vi "PicoLog_main.vi"() -> ()   [LabVIEW 2014]
uses:
  picohrdl.dll
panel:
  in  "Save?":bool=TRUE caption="Save"
  out "noOfOpen\nChannels":i16=1
  out "Ch nr. 14":string[](array[string])
  out "Ch nr. 13":string[](array[string])
  out "Ch nr. 12":string[](array[string])
  out "Ch nr. 11":string[](array[string])
  out "Ch nr. 10":string[](array[string])
  out "Ch nr. 9":string[](array[string])
  out "Ch nr. 8":string[](array[string])
  out "Ch nr. 7":string[](array[string])
  out "Ch nr. 6":string[](array[string])
  out "Ch nr. 5":string[](array[string])
  out "Ch nr. 4":string[](array[string])
  out "Ch nr. 3":string[](array[string])
  out "Ch nr. 2.35":string[](array[string])
  out "Ch nr. 2":string[](array[string])
  out "Ch nr. 1":string[](array[string])
  out "Ch nr. 0":string[](array[string])=["1", "8"]
  out "P1 17":dbl[](graph)
  out "P1 16":dbl[](graph)
  out "P1 15":dbl[](graph)
  out "P1 14":dbl[](graph)
  out "P1 13":dbl[](graph)
  out "P1 12":dbl[](graph)
  out "P1 11":dbl[](graph)
  out "P1 10":dbl[](graph)
  out "P1 9":dbl[](graph)
  out "P1 8":dbl[](graph)
  out "P1 7":dbl[](graph)
  out "P1 6":dbl[](graph)
  out "P1 5":dbl[](graph)
  out "P1 4":dbl[](graph)
  out "P1 3":dbl[](graph)
  out "P1 2":dbl[](graph)
  in  "Voltage range":i32[](array[numeric])=[0, 0, 0, 0, 0, 0, 0, 0, 0, 0, 0, 0, 0, 0, 0, 0] min=0 max=6 step=1
  in  "Single ended\n(1- single)\n(0 - difer)":i32[](array[numeric])=[1, 1, 1, 1, 1, 1, 1, 1, 1, 1, 1, 1, 1, 1, 1, 1] min=0 max=1 step=1
  in  "Ch nr":bool[](array[boolean])=[FALSE, FALSE, FALSE, FALSE, FALSE, FALSE, FALSE, FALSE, FALSE, FALSE, FALSE, FALSE, FALSE, FALSE, FALSE, FALSE]
  in  "conversionTime":i16(ring)=3 items=["60 ms", "100 ms", "180 ms", "340 ms", "660 ms"]
  in  "Mains Frequency":i16(ring) items=["50 Hz", "60 Hz"]
  in  "sampleInterval_ms":i32=1000
  in  "stop":bool
  # "1       2       3      4       5        6       7       8       9      10     11      12     13    14       15     16"
  # "0 -+2500mV\n1 -+1250mV\n2 -+625mV\n3 -+313mV\n4 -+156mV\n5 -+78mv\n6 -+39mV"
  # "Channel"
  # "Channel"
  # "Channel"
  # "Channel"
  # "Channel"
  # "Channel"
  # "Channel"
  # "Channel"
  # "Channel"
  # "Channel"
  # "Channel"
  # "Channel"
  # "Channel"
  # "Channel"
  # "Channel"
  # "Channel"
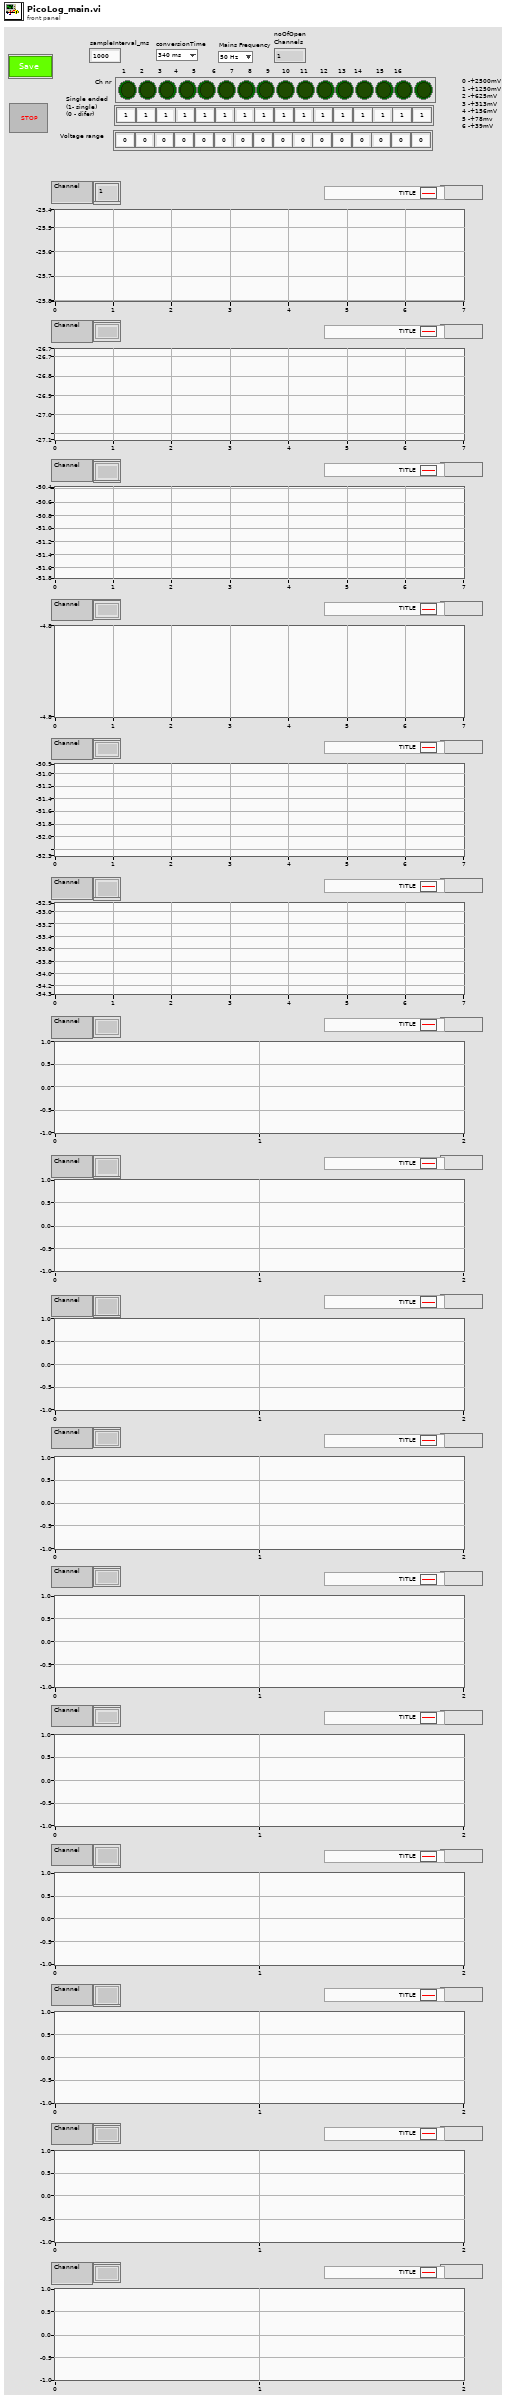
[diagram p1: front panel]
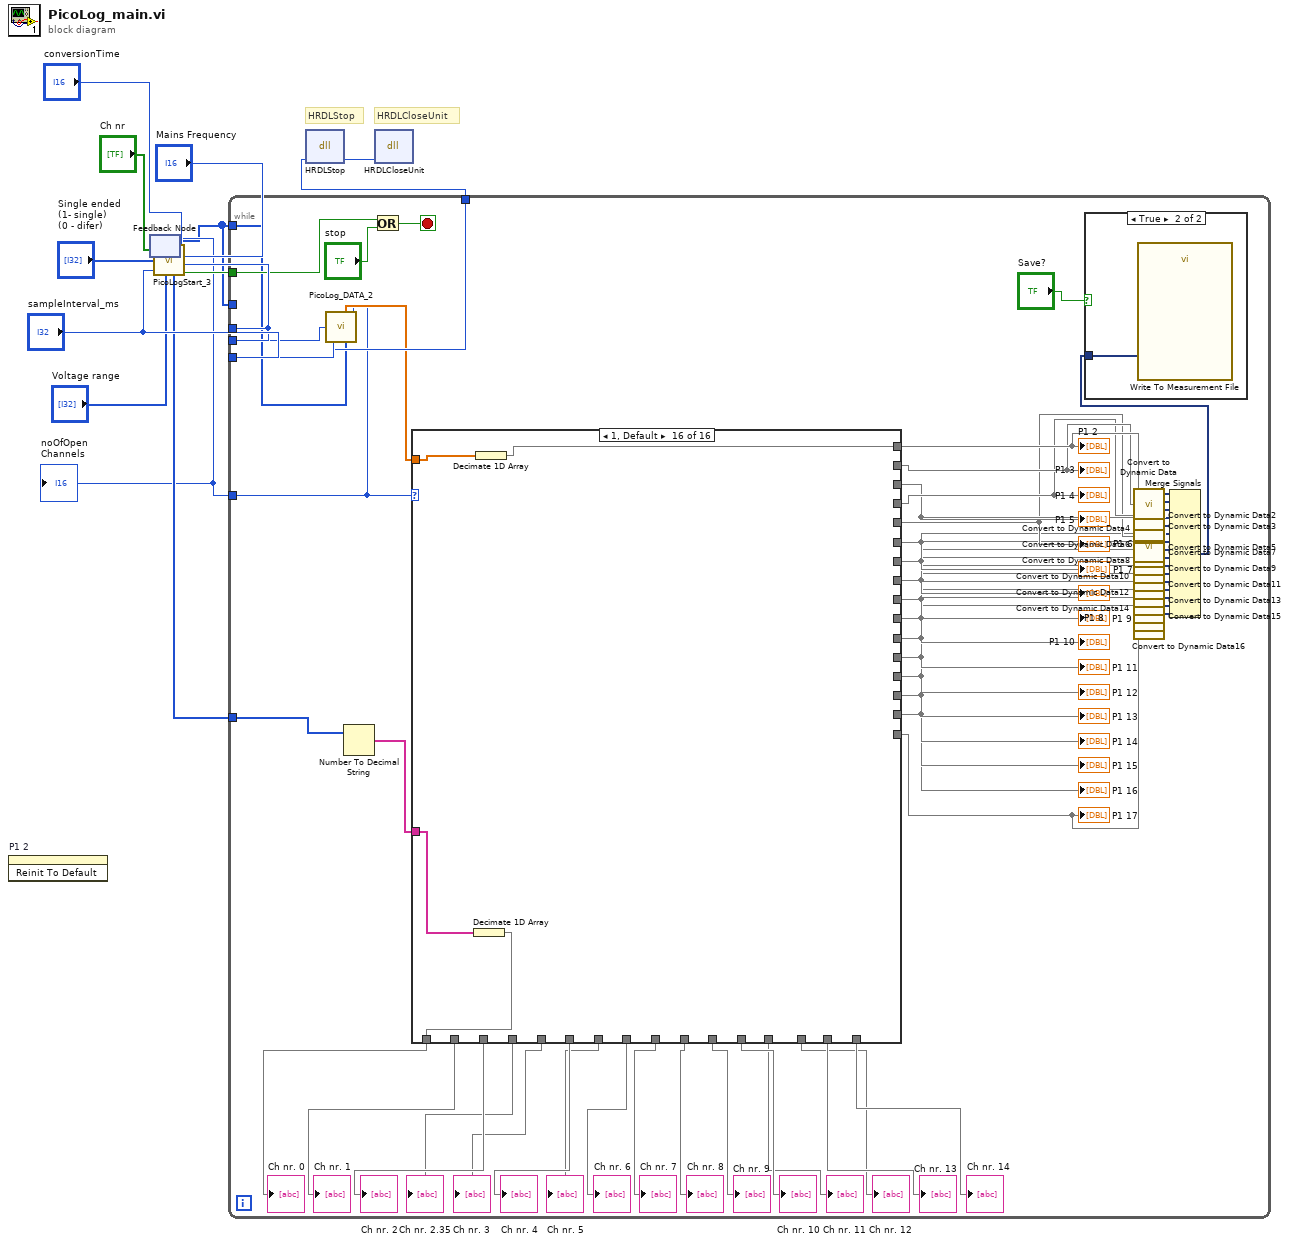
[diagram p0: block diagram]
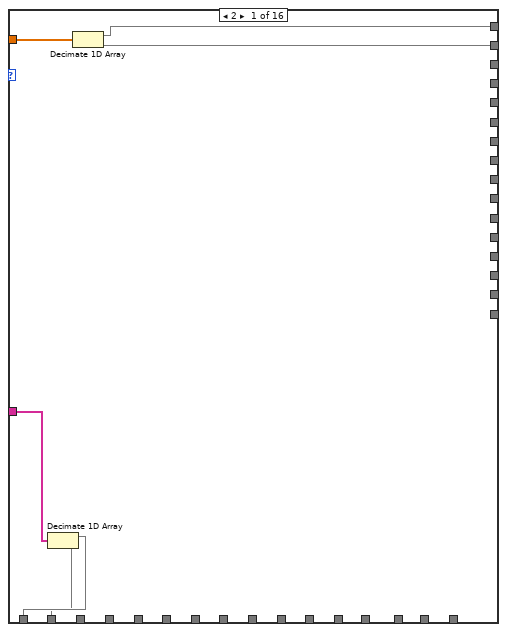
[diagram p3: hidden frame]
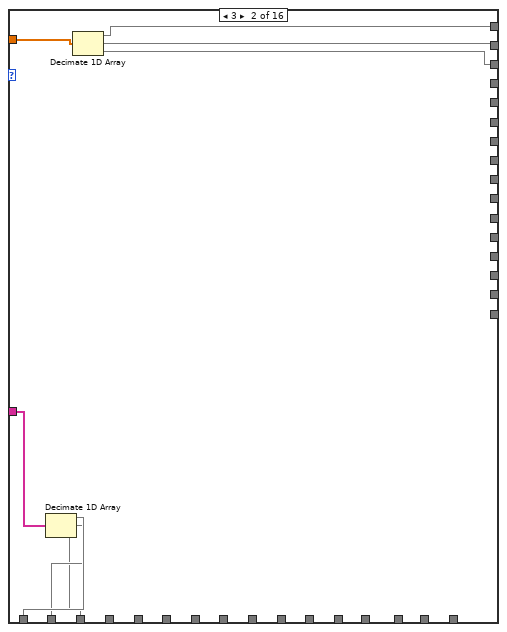
[diagram p4: hidden frame]
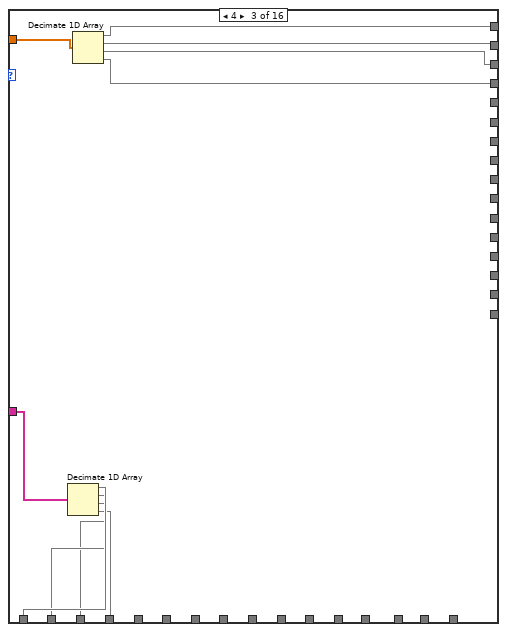
[diagram p5: hidden frame]
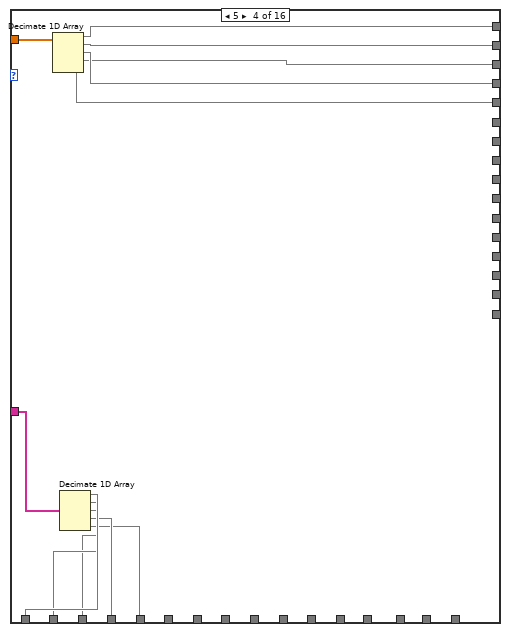
[diagram p6: hidden frame]
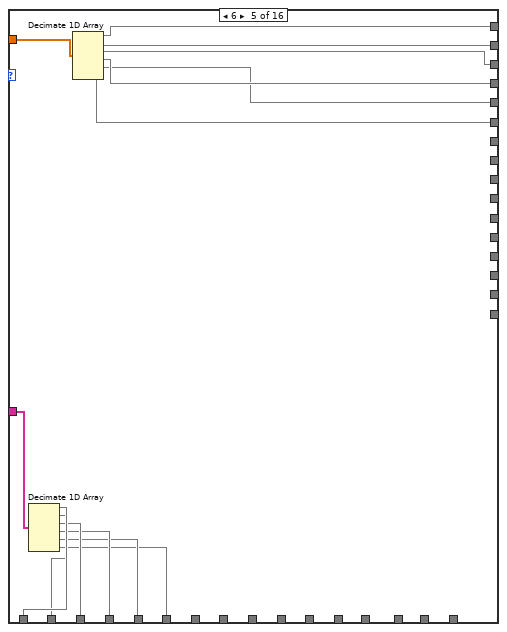
[diagram p7: hidden frame]
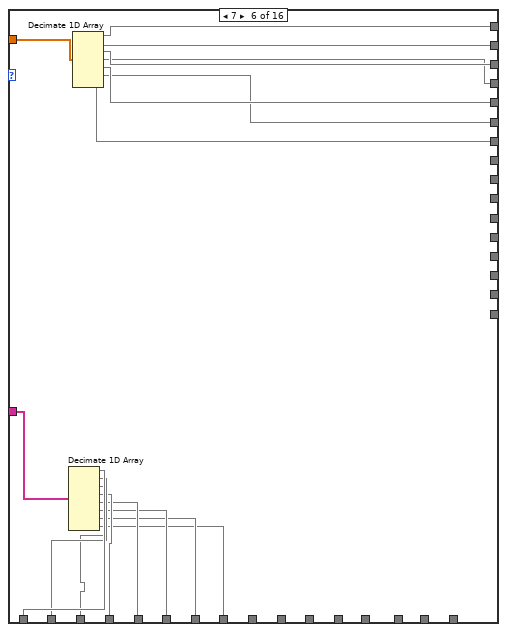
[diagram p8: hidden frame]
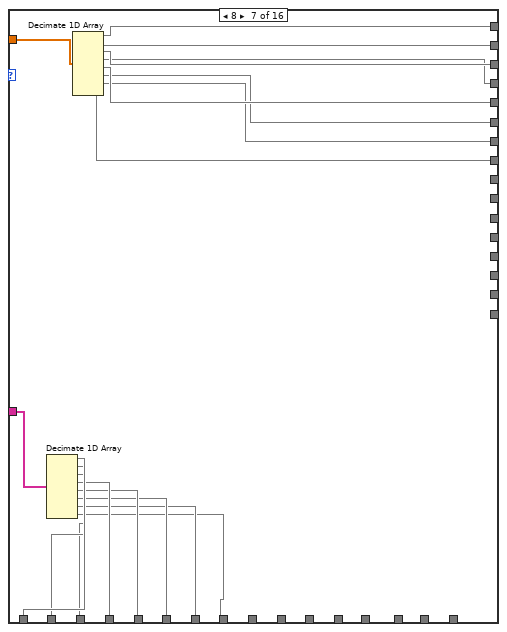
[diagram p9: hidden frame]
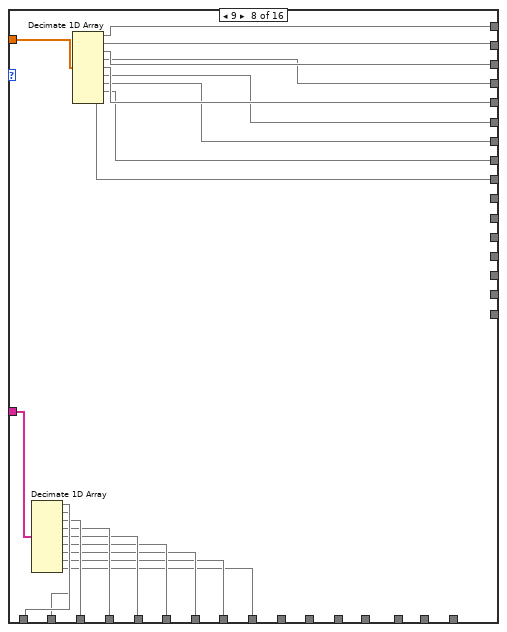
[diagram p10: hidden frame]
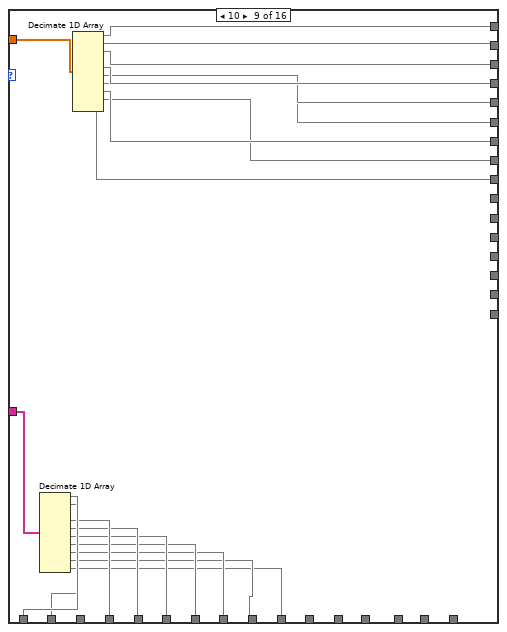
[diagram p11: hidden frame]
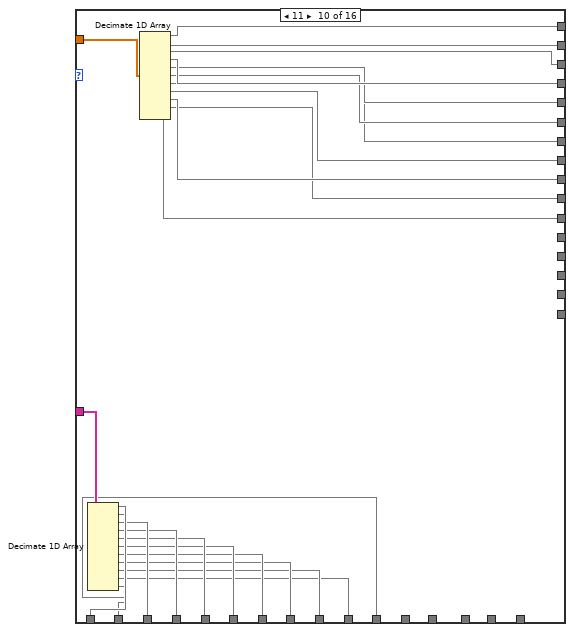
[diagram p12: hidden frame]
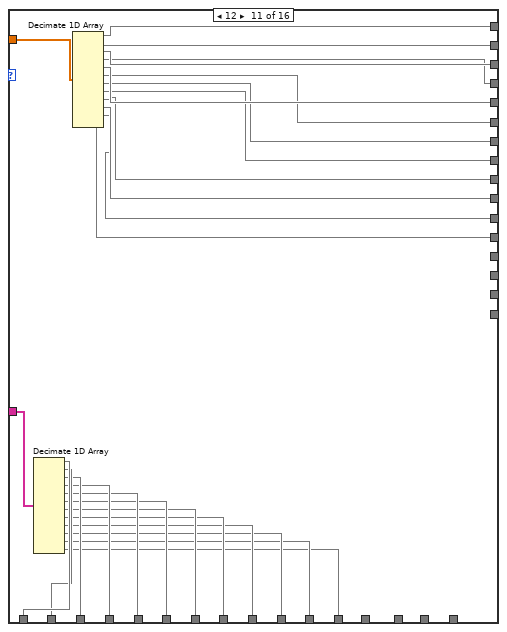
[diagram p13: hidden frame]
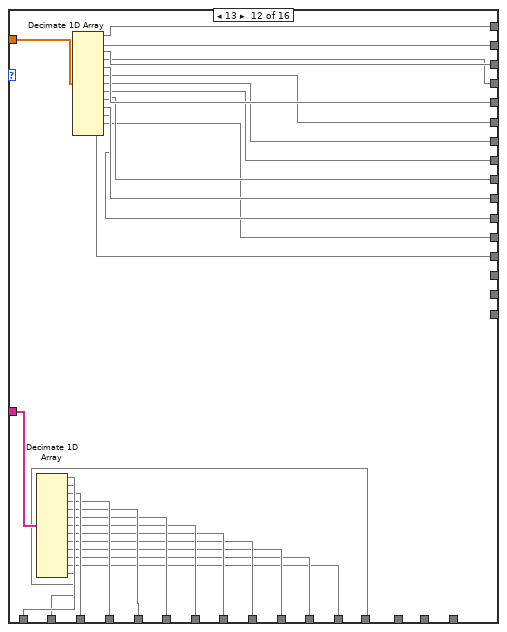
[diagram p14: hidden frame]
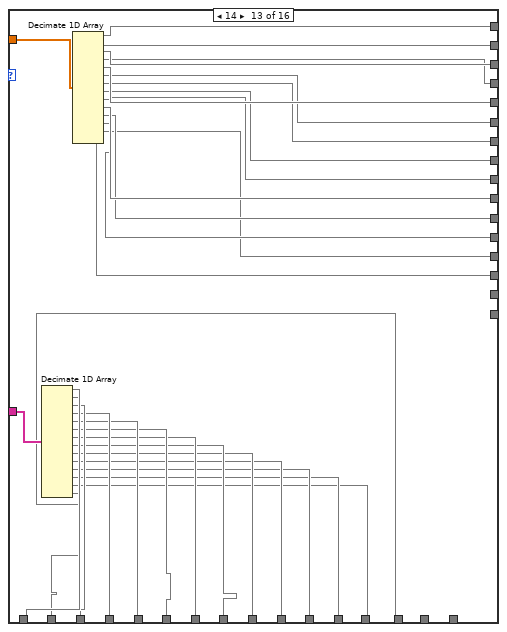
[diagram p15: hidden frame]
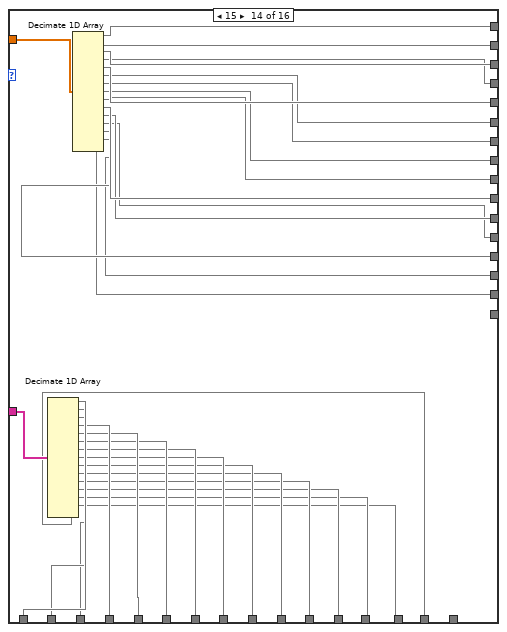
[diagram p16: hidden frame]
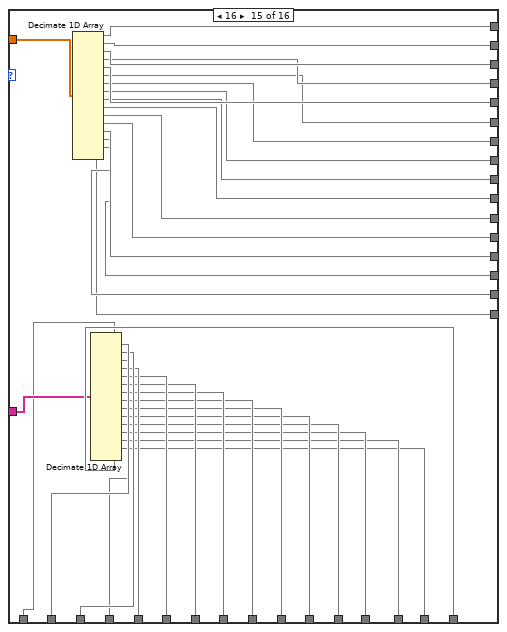
[diagram p17: hidden frame]
diagram:
  # "HRDLStop"
  # "HRDLCloseUnit"
  n1 = invoke on="P1 2" class="WFChart (strict)" method="Reinit To Default"() -> ()  [unwired: 3 in, 3 out]
  n2 = feedback #1() -> (w1:i32[])  [unwired: 1 in]
  n3 = call "PicoLogStart_3.vi"("Ch nr"="Ch nr", "Single ended\n(0- single)\n(1 - difer)"="Single ended\n(1- single)\n(0 - difer)", "sampleInterval_ms"="sampleInterval_ms", "Voltage range"="Voltage range", "conversionTime"="conversionTime", "Mains Frequency"="Mains Frequency") -> ("Voltage range"=w2:i32[], "noOfChannels"=w4:i16, "ChNrSkArr"=w5:i32[], "handle"=w6:i16, "STOP"=w8:bool)
  "noOfOpen\nChannels" <- w4
  n4 = feedback-in #1(w2) -> ()
  n5 = while {
    tunnel: w6 -> [_]
    tunnel: "sampleInterval_ms" -> [w71]
    tunnel: w8 -> [w73]
    tunnel: [w70] -> w3
    tunnel: w1 -> [_]
    tunnel: w6 -> [w72]
    tunnel: w5 -> [w52]
    tunnel: w4 -> [w50]
    tunnel: w1 -> [w15]
    stop <- w75 stop-if-true
    n6 = call "PicoLog_DATA_2.vi"("k m"=w15, "noOfChannels"=w50, "handle"=w72, "sampleInterval_ms"=w71) -> ("x*y"=w51:dbl[], "handle"=w70:i16)  [unwired: 3 in]
    n7 = Number To Decimal String(number=w52) -> (decimal integer string=w68:string[])  [unwired: 1 in]
    n8 = Or(x=w73, y="stop") -> (x .or. y?=w75:bool)
    n9 = case shown="1, Default" w50 {
      tunnel: w51 -> [w82 w90 w100 w112 w126 w143 w161 w181 w201 w225 w251 w279 w309 w341 w375 w379]
      tunnel: [w81 w89 w99 w111 w125 w142 w160 w180 w200 w224 w250 w278 w308 w340 w374 w378] -> w47
      tunnel: [w80 w88 w98 w110 w124 w141 w159 w179 w199 w223 w249 w277 w307 w339 w373 _] -> w45
      tunnel: [_ _ w96 w109 w122 w139 w157 w177 w197 w222 w247 w275 w305 w337 w371 _] -> w43
      tunnel: [_ w87 w97 w108 w123 w140 w158 w178 w198 w221 w248 w276 w306 w338 w372 _] -> w41
      tunnel: [_ _ _ w107 w121 w138 w156 w176 w196 w220 w246 w274 w304 w336 w370 _] -> w39
      tunnel: [_ _ _ _ w120 w137 w155 w175 w195 w219 w245 w273 w303 w335 w369 _] -> w37
      tunnel: [_ _ _ _ _ w136 w154 w174 w194 w218 w244 w272 w302 w334 w368 _] -> w35
      tunnel: [_ _ _ _ _ _ w153 w173 w193 w217 w243 w271 w301 w333 w367 _] -> w33
      tunnel: [_ _ _ _ _ _ _ w172 w192 w216 w242 w270 w300 w332 w366 _] -> w31
      tunnel: [_ _ _ _ _ _ _ _ _ w215 w241 w269 w299 w331 w365 _] -> w29
      tunnel: [_ _ _ _ _ _ _ _ _ w214 w240 w268 w298 w330 w364 _] -> w27
      tunnel: [_ _ _ _ _ _ _ _ _ _ w239 w267 w297 w329 w363 _] -> w25
      tunnel: [_ _ _ _ _ _ _ _ _ _ _ w266 w296 w328 w362 _] -> w23
      tunnel: [_ _ _ _ _ _ _ _ _ _ _ _ w295 w327 w361 _] -> w21
      tunnel: [_ _ _ _ _ _ _ _ _ _ _ _ _ w326 w360 _] -> w19
      tunnel: [_ _ _ _ _ _ _ _ _ _ _ _ _ _ w359 _] -> w17
      tunnel: [_ _ _ _ _ _ _ _ _ _ _ _ _ _ w358 _] -> w69
      tunnel: w68 -> [w79 w86 w95 w106 w119 w135 w152 w171 w191 w213 w238 w265 w294 w325 w357 w377]
      tunnel: [w78 w85 w94 w105 w118 w134 w151 w170 w190 w212 w237 w264 w293 w324 w356 w376] -> w67
      tunnel: [_ _ _ _ _ _ _ _ _ _ _ _ _ w310 w342 _] -> w66
      tunnel: [w77 w84 w93 w104 w117 w133 w150 w169 w189 w211 w236 w263 w292 w323 w355 _] -> w65
      tunnel: [_ w83 w92 w103 w116 w132 w149 w168 _ w210 w235 w262 w291 w322 w354 _] -> w64
      tunnel: [_ _ w91 w102 w115 w131 w148 w167 w188 w209 w234 w261 w290 w321 w353 _] -> w63
      tunnel: [_ _ _ w101 w114 w130 w147 w166 w187 w208 w233 w260 w289 w320 w352 _] -> w53
      tunnel: [_ _ _ _ w113 w129 w146 w165 w186 w207 w232 w259 w288 w319 w351 _] -> w62
      tunnel: [_ _ _ _ _ w128 w145 w164 w185 w206 w231 w258 w287 w318 w350 _] -> w61
      tunnel: [_ _ _ _ _ w127 w144 w163 w184 w205 w230 w257 w286 w317 w349 _] -> w60
      tunnel: [_ _ _ _ _ _ _ w162 w183 w204 w229 w256 w285 w316 w348 _] -> w59
      tunnel: [_ _ _ _ _ _ _ _ w182 w203 w228 w255 w284 w315 w347 _] -> w58
      tunnel: [_ _ _ _ _ _ _ _ _ w202 w227 w254 w283 w314 w346 _] -> w57
      tunnel: [_ _ _ _ _ _ _ _ _ _ w226 w253 w282 w313 w345 _] -> w56
      tunnel: [_ _ _ _ _ _ _ _ _ _ _ w252 w281 w312 w344 _] -> w55
      tunnel: [_ _ _ _ _ _ _ _ _ _ _ _ w280 w311 w343 _] -> w54
      frame 2 {
        n10 = Decimate 1D Array(w79) -> (w78:string[], w77:string[])
        n11 = Decimate 1D Array(w82) -> (w81:dbl[], w80:dbl[])
      }
      frame 3 {
        n12 = Decimate 1D Array(w86) -> (w85:string[], w84:string[], w83:string[])
        n13 = Decimate 1D Array(w90) -> (w89:dbl[], w88:dbl[], w87:dbl[])
      }
      frame 4 {
        n14 = Decimate 1D Array(w95) -> (w94:string[], w93:string[], w92:string[], w91:string[])
        n15 = Decimate 1D Array(w100) -> (w99:dbl[], w98:dbl[], w97:dbl[], w96:dbl[])
      }
      frame 5 {
        n16 = Decimate 1D Array(w112) -> (w111:dbl[], w110:dbl[], w109:dbl[], w108:dbl[], w107:dbl[])
        n17 = Decimate 1D Array(w106) -> (w105:string[], w104:string[], w103:string[], w102:string[], w101:string[])
      }
      frame 6 {
        n18 = Decimate 1D Array(w119) -> (w118:string[], w117:string[], w116:string[], w115:string[], w114:string[], w113:string[])
        n19 = Decimate 1D Array(w126) -> (w125:dbl[], w124:dbl[], w123:dbl[], w122:dbl[], w121:dbl[], w120:dbl[])
      }
      frame 7 {
        n20 = Decimate 1D Array(w135) -> (w134:string[], w133:string[], w132:string[], w131:string[], w130:string[], w129:string[], w128:string[], w127:string[])
        n21 = Decimate 1D Array(w143) -> (w142:dbl[], w141:dbl[], w140:dbl[], w139:dbl[], w138:dbl[], w137:dbl[], w136:dbl[])
      }
      frame 8 {
        n22 = Decimate 1D Array(w152) -> (w151:string[], w150:string[], w149:string[], w148:string[], w147:string[], w146:string[], w145:string[], w144:string[])
        n23 = Decimate 1D Array(w161) -> (w160:dbl[], w159:dbl[], w158:dbl[], w157:dbl[], w156:dbl[], w155:dbl[], w154:dbl[], w153:dbl[])
      }
      frame 9 {
        n24 = Decimate 1D Array(w171) -> (w170:string[], w169:string[], w168:string[], w167:string[], w166:string[], w165:string[], w164:string[], w163:string[], w162:string[])
        n25 = Decimate 1D Array(w181) -> (w180:dbl[], w179:dbl[], w178:dbl[], w177:dbl[], w176:dbl[], w175:dbl[], w174:dbl[], w173:dbl[], w172:dbl[])
      }
      frame 10 {
        n26 = Decimate 1D Array(w191) -> (w190:string[], w189:string[], w188:string[], w187:string[], w186:string[], w185:string[], w184:string[], w183:string[], w182:string[])  [unwired: 1 out]
        n27 = Decimate 1D Array(w201) -> (w200:dbl[], w199:dbl[], w198:dbl[], w197:dbl[], w196:dbl[], w195:dbl[], w194:dbl[], w193:dbl[], w192:dbl[])  [unwired: 1 out]
      }
      frame 11 {
        n28 = Decimate 1D Array(w213) -> (w212:string[], w211:string[], w210:string[], w209:string[], w208:string[], w207:string[], w206:string[], w205:string[], w204:string[], w203:string[], w202:string[])
        n29 = Decimate 1D Array(w225) -> (w224:dbl[], w223:dbl[], w221:dbl[], w222:dbl[], w220:dbl[], w219:dbl[], w218:dbl[], w217:dbl[], w216:dbl[], w215:dbl[], w214:dbl[])
      }
      frame 12 {
        n30 = Decimate 1D Array(w238) -> (w237:string[], w236:string[], w235:string[], w234:string[], w233:string[], w232:string[], w231:string[], w230:string[], w229:string[], w228:string[], w227:string[], w226:string[])
        n31 = Decimate 1D Array(w251) -> (w250:dbl[], w249:dbl[], w248:dbl[], w247:dbl[], w246:dbl[], w245:dbl[], w244:dbl[], w243:dbl[], w242:dbl[], w241:dbl[], w240:dbl[], w239:dbl[])
      }
      frame 13 {
        n32 = Decimate 1D Array(w265) -> (w264:string[], w263:string[], w262:string[], w261:string[], w260:string[], w259:string[], w258:string[], w257:string[], w256:string[], w255:string[], w254:string[], w253:string[], w252:string[])
        n33 = Decimate 1D Array(w279) -> (w278:dbl[], w277:dbl[], w276:dbl[], w275:dbl[], w274:dbl[], w273:dbl[], w272:dbl[], w271:dbl[], w270:dbl[], w269:dbl[], w268:dbl[], w267:dbl[], w266:dbl[])
      }
      frame 14 {
        n34 = Decimate 1D Array(w294) -> (w293:string[], w292:string[], w291:string[], w290:string[], w289:string[], w288:string[], w287:string[], w286:string[], w285:string[], w284:string[], w283:string[], w282:string[], w281:string[], w280:string[])
        n35 = Decimate 1D Array(w309) -> (w308:dbl[], w307:dbl[], w306:dbl[], w305:dbl[], w304:dbl[], w303:dbl[], w302:dbl[], w301:dbl[], w300:dbl[], w299:dbl[], w298:dbl[], w297:dbl[], w296:dbl[], w295:dbl[])
      }
      frame 15 {
        n36 = Decimate 1D Array(w325) -> (w324:string[], w323:string[], w322:string[], w321:string[], w320:string[], w319:string[], w318:string[], w317:string[], w316:string[], w315:string[], w314:string[], w313:string[], w312:string[], w311:string[], w310:string[])
        n37 = Decimate 1D Array(w341) -> (w340:dbl[], w339:dbl[], w338:dbl[], w337:dbl[], w336:dbl[], w335:dbl[], w334:dbl[], w333:dbl[], w332:dbl[], w331:dbl[], w330:dbl[], w329:dbl[], w328:dbl[], w327:dbl[], w326:dbl[])
      }
      frame 16 {
        n38 = Decimate 1D Array(w375) -> (w374:dbl[], w373:dbl[], w372:dbl[], w371:dbl[], w370:dbl[], w369:dbl[], w368:dbl[], w367:dbl[], w366:dbl[], w365:dbl[], w364:dbl[], w363:dbl[], w362:dbl[], w361:dbl[], w360:dbl[], w359:dbl[])
        n39 = Decimate 1D Array(w357) -> (w356:string[], w355:string[], w354:string[], w353:string[], w352:string[], w351:string[], w350:string[], w349:string[], w348:string[], w347:string[], w346:string[], w345:string[], w344:string[], w343:string[], w342:string[], w358:string[])
      }
      frame 1, Default {
        n40 = Decimate 1D Array(w377) -> (w376:string[])
        n41 = Decimate 1D Array(w379) -> (w378:dbl[])
      }
    }
    "P1 2" <- w47
    "P1 3" <- w45
    "P1 4" <- w43
    "P1 5" <- w41
    "P1 6" <- w39
    "P1 7" <- w37
    "P1 8" <- w35
    "P1 9" <- w33
    "P1 10" <- w31
    "P1 11" <- w29
    "P1 12" <- w27
    "P1 13" <- w25
    "P1 14" <- w23
    "P1 15" <- w21
    "P1 16" <- w19
    "P1 17" <- w17
    "Ch nr. 0" <- w67
    "Ch nr. 1" <- w65
    "Ch nr. 2" <- w64
    "Ch nr. 2.35" <- w63
    "Ch nr. 3" <- w53
    "Ch nr. 4" <- w62
    "Ch nr. 5" <- w61
    "Ch nr. 6" <- w60
    "Ch nr. 7" <- w59
    "Ch nr. 8" <- w58
    "Ch nr. 9" <- w57
    "Ch nr. 10" <- w56
    "Ch nr. 11" <- w55
    "Ch nr. 12" <- w54
    "Ch nr. 13" <- w66
    "Ch nr. 14" <- w69
    n42 = call "Convert to Dynamic Data"("Array"=w47) -> ("Dynamic Data Type"=w46:dynamicdata)  [unwired: 3 in]
    n43 = call "Convert to Dynamic Data2"("Array"=w45) -> ("Dynamic Data Type"=w44:dynamicdata)  [unwired: 3 in]
    n44 = call "Convert to Dynamic Data3"("Array"=w43) -> ("Dynamic Data Type"=w42:dynamicdata)  [unwired: 3 in]
    n45 = call "Convert to Dynamic Data4"("Array"=w41) -> ("Dynamic Data Type"=w40:dynamicdata)  [unwired: 3 in]
    n46 = call "Convert to Dynamic Data6"("Array"=w37) -> ("Dynamic Data Type"=w36:dynamicdata)  [unwired: 3 in]
    n47 = call "Convert to Dynamic Data5"("Array"=w39) -> ("Dynamic Data Type"=w38:dynamicdata)  [unwired: 3 in]
    n48 = call "Convert to Dynamic Data7"("Array"=w35) -> ("Dynamic Data Type"=w34:dynamicdata)  [unwired: 3 in]
    n49 = call "Convert to Dynamic Data8"("Array"=w33) -> ("Dynamic Data Type"=w32:dynamicdata)  [unwired: 3 in]
    n50 = call "Convert to Dynamic Data9"("Array"=w31) -> ("Dynamic Data Type"=w30:dynamicdata)  [unwired: 3 in]
    n51 = call "Convert to Dynamic Data10"("Array"=w29) -> ("Dynamic Data Type"=w28:dynamicdata)  [unwired: 3 in]
    n52 = call "Convert to Dynamic Data11"("Array"=w27) -> ("Dynamic Data Type"=w26:dynamicdata)  [unwired: 3 in]
    n53 = call "Convert to Dynamic Data12"("Array"=w25) -> ("Dynamic Data Type"=w24:dynamicdata)  [unwired: 3 in]
    n54 = call "Convert to Dynamic Data13"("Array"=w23) -> ("Dynamic Data Type"=w22:dynamicdata)  [unwired: 3 in]
    n55 = call "Convert to Dynamic Data14"("Array"=w21) -> ("Dynamic Data Type"=w20:dynamicdata)  [unwired: 3 in]
    n56 = call "Convert to Dynamic Data15"("Array"=w19) -> ("Dynamic Data Type"=w18:dynamicdata)  [unwired: 3 in]
    n57 = call "Convert to Dynamic Data16"("Array"=w17) -> ("Dynamic Data Type"=w16:dynamicdata)  [unwired: 3 in]
    n58 = Merge Signals(w46, w44, w42, w40, w38, w36, w34, w32, w30, w28, w26, w24, w22, w20, w18, w16) -> (w48:dynamicdata)
    n59 = case shown="True" "Save?" {
      tunnel: w48 -> [_ w76]
      frame False {
      }
      frame True {
        n60 = call "Write To Measurement File"("Signals"=w76) -> ()  [unwired: 16 in, 3 out]
      }
    }
  }
  n61 = dll-call lib="picohrdl.dll" fn="HRDLStop"("handle"=w3) -> ("handle"=w14:i16)  [unwired: 4 in, 2 out]
  n62 = dll-call lib="PicoHRDL.dll" fn="HRDLCloseUnit"("handle"=w14) -> ()  [unwired: 5 in, 2 out]
